vi "Main.vi"(8 "error in (no error)":errorcluster, 11 "AOTFBase in":refnum<class "AOTF.lvclass">) -> (0 "error out":errorcluster, 3 "component":refnum<class "AOTF.lvclass">)   [LabVIEW 2012, in "AOTF.lvclass"]
doc: "Main VI of the component."
uses:
  AOTF.lvclass
  <vilib>/Distrio/Murmex/Murmex/command_enum.ctl
  Controls/laser line ring.ctl
  <vilib>/Distrio/Murmex/InitialiseMessage/InitialiseMessage.lvclass
  AOTF.lvclass/AOTF.ctl
  <vilib>/Distrio/Murmex/ConfigureMessage/ConfigureMessage.lvclass
  <vilib>/Distrio/Murmex/TerminateMessage/TerminateMessage.lvclass
  <vilib>/Distrio/Murmex/Murmex/update_cluster.ctl
  <vilib>/Distrio/Murmex/Murmex/Set configure at initialise.vi
  <vilib>/Distrio/Murmex/Murmex/Set VI reference.vi
  <vilib>/Distrio/Murmex/Murmex/Get ID.vi
  <vilib>/Distrio/Murmex/Murmex/Set log reference.vi
  <vilib>/Distrio/Murmex/Murmex/Murmex.lvclass
  <vilib>/Distrio/Murmex/Message/Message.lvclass
panel:
  in  "button::configure":bool
  in  "button::quit":bool
  out "terminate?":bool=TRUE
  in  "Tab Control":enum32{"Main", "Debug"}(tab)
  in  "Power":dbl(knob) caption="Power [%]" min=0.0 max=100.0 scale=0.0..100.0
  in  "Wavelength":T1=10 items=["Blind"=10, "405nm"=0, "445nm"=5, "491nm"=1, "515nm"=2, "561nm"=3]
  out "log":string="\r\n11:11:41.970 05/12/2013: initialise from AOTF to AOTF\r\n11:11:42.586 05/12/2013: inform from AOTF to AOTF\r\n11:11:43.913 05/12/2013: update from AOTF to AOTF\r\n11:11:45.142 05/12/2013: generic (shutter_off) from AOTF to AOTF\r\n11:11:45.270 05/12/2013: generic (shutter_on) from AOTF to AOTF\r\n11:11:45.902 05/12/2013: generic (shutter_off) from AOTF to AOTF\r\n11:11:45.932 05/12/2013: inspect from AOTF to AOTF\r\n11:11:48.013 05/12/2013: configure from AOTF to AOTF\r\n11:11:52.003 05/12/2013: inform from AOTF to AOTF\r\n11:11:58.521 05/12/2013: initialise from AOTF to AOTF\r\n11:11:58.561 05/12/2013: inform from AOTF to AOTF\r\n11:11:58.695 05/12/2013: inform from AOTF to AOTF\r\n11:12:02.089 05/12/2013: update from AOTF to AOTF\r\n11:12:02.308 05/12/2013: inspect from AOTF to AOTF\r\n11:12:02.364 05/12/2013: inform from AOTF to AOTF\r\n11:12:05.062 05/12/2013: generic (shutter_on) from AOTF to AOTF\r\n11:12:06.690 05/12/2013: update from AOTF to AOTF\r\n11:12:06.909 05/12/2013: inspect from AOTF to AOTF\r\n11:12:06.964 05/12/2013: inform from AOTF to AOTF\r\n11:12:07.770 05/12/2013: update from AOTF to AOTF\r\n11:12:07.989 05/12/2013: inspect from AOTF to AOTF\r\n11:12:08.044 05/12/2013: inform from AOTF to AOTF\r\n11:12:08.627 05/12/2013: update from AOTF to AOTF\r\n11:12:08.846 05/12/2013: inspect from AOTF to AOTF\r\n11:12:08.900 05/12/2013: inform from AOTF to AOTF\r\n11:12:09.290 05/12/2013: update from AOTF to AOTF\r\n11:12:09.508 05/12/2013: inspect from AOTF to AOTF\r\n11:12:09.563 05/12/2013: inform from AOTF to AOTF\r\n11:12:10.154 05/12/2013: update from AOTF to AOTF\r\n11:12:10.373 05/12/2013: inspect from AOTF to AOTF\r\n11:12:10.430 05/12/2013: inform from AOTF to AOTF\r\n11:12:20.953 05/12/2013: update from AOTF to AOTF\r\n11:12:21.172 05/12/2013: inspect from AOTF to AOTF\r\n11:12:21.227 05/12/2013: inform from AOTF to AOTF\r\n11:12:22.057 05/12/2013: update from AOTF to AOTF\r\n11:12:22.276 05/12/2013: inspect from AOTF to AOTF\r\n11:12:22.330 05/12/2013: inform from AOTF to AOTF\r\n11:12:22.841 05/12/2013: update from AOTF to AOTF\r\n11:12:23.060 05/12/2013: inspect from AOTF to AOTF\r\n11:12:23.114 05/12/2013: inform from AOTF to AOTF\r\n11:12:23.449 05/12/2013: update from AOTF to AOTF\r\n11:12:23.668 05/12/2013: inspect from AOTF to AOTF\r\n11:12:23.724 05/12/2013: inform from AOTF to AOTF\r\n11:12:24.514 05/12/2013: update from AOTF to AOTF\r\n11:12:24.733 05/12/2013: inspect from AOTF to AOTF\r\n11:12:24.789 05/12/2013: inform from AOTF to AOTF\r\n11:12:25.098 05/12/2013: update from AOTF to AOTF\r\n11:12:25.317 05/12/2013: inspect from AOTF to AOTF\r\n11:12:25.371 05/12/2013: inform from AOTF to AOTF\r\n11:12:26.482 05/12/2013: update from AOTF to AOTF\r\n11:12:26.701 05/12/2013: inspect from AOTF to AOTF\r\n11:12:26.755 05/12/2013: inform from AOTF to AOTF\r\n11:12:27.154 05/12/2013: update from AOTF to AOTF\r\n11:12:27.373 05/12/2013: inspect from AOTF to AOTF\r\n11:12:27.428 05/12/2013: inform from AOTF to AOTF\r\n11:12:27.666 05/12/2013: update from AOTF to AOTF\r\n11:12:27.885 05/12/2013: inspect from AOTF to AOTF\r\n11:12:27.944 05/12/2013: inform from AOTF to AOTF\r\n11:12:33.380 05/12/2013: update from AOTF to AOTF\r\n11:12:33.484 05/12/2013: update from AOTF to AOTF\r\n11:12:33.603 05/12/2013: inspect from AOTF to AOTF\r\n11:12:33.611 05/12/2013: update from AOTF to AOTF\r\n11:12:33.684 05/12/2013: update from AOTF to AOTF\r\n11:12:33.740 05/12/2013: update from AOTF to AOTF\r\n11:12:33.827 05/12/2013: inspect from AOTF to AOTF\r\n11:12:33.835 05/12/2013: update from AOTF to AOTF\r\n11:12:33.897 05/12/2013: inform from AOTF to AOTF\r\n11:12:33.903 05/12/2013: update from AOTF to AOTF\r\n11:12:33.940 05/12/2013: update from AOTF to AOTF\r\n11:12:34.085 05/12/2013: update from AOTF to AOTF\r\n11:12:34.119 05/12/2013: inspect from AOTF to AOTF\r\n11:12:34.292 05/12/2013: update from AOTF to AOTF\r\n11:12:34.336 05/12/2013: inspect from AOTF to AOTF\r\n11:12:34.553 05/12/2013: inspect from AOTF to AOTF\r\n11:12:34.608 05/12/2013: inform from AOTF to AOTF\r\n11:12:34.739 05/12/2013: update from AOTF to AOTF\r\n11:12:34.771 05/12/2013: update from AOTF to AOTF\r\n11:12:34.826 05/12/2013: inspect from AOTF to AOTF\r\n11:12:34.834 05/12/2013: update from AOTF to AOTF\r\n11:12:34.867 05/12/2013: update from AOTF to AOTF\r\n11:12:34.931 05/12/2013: update from AOTF to AOTF\r\n11:12:34.979 05/12/2013: update from AOTF to AOTF\r\n11:12:35.003 05/12/2013: update from AOTF to AOTF\r\n11:12:35.027 05/12/2013: update from AOTF to AOTF\r\n11:12:35.041 05/12/2013: update from AOTF to AOTF\r\n11:12:35.051 05/12/2013: inspect from AOTF to AOTF\r\n11:12:35.066 05/12/2013: update from AOTF to AOTF\r\n11:12:35.116 05/12/2013: update from AOTF to AOTF\r\n11:12:35.171 05/12/2013: update from AOTF to AOTF\r\n11:12:35.211 05/12/2013: update from AOTF to AOTF\r\n11:12:35.273 05/12/2013: inspect from AOTF to AOTF\r\n11:12:35.287 05/12/2013: update from AOTF to AOTF\r\n11:12:35.475 05/12/2013: update from AOTF to AOTF\r\n11:12:35.495 05/12/2013: inspect from AOTF to AOTF\r\n11:12:35.549 05/12/2013: inform from AOTF to AOTF\r\n11:12:35.764 05/12/2013: inspect from AOTF to AOTF\r\n11:12:35.819 05/12/2013: inform from AOTF to AOTF\r\n11:12:35.861 05/12/2013: update from AOTF to AOTF\r\n11:12:35.877 05/12/2013: inform from AOTF to AOTF\r\n11:12:35.947 05/12/2013: update from AOTF to AOTF\r\n11:12:36.067 05/12/2013: update from AOTF to AOTF\r\n11:12:36.100 05/12/2013: inspect from AOTF to AOTF\r\n11:12:36.235 05/12/2013: update from AOTF to AOTF\r\n11:12:36.317 05/12/2013: inspect from AOTF to AOTF\r\n11:12:36.371 05/12/2013: inform from AOTF to AOTF\r\n11:12:36.587 05/12/2013: inspect from AOTF to AOTF\r\n11:12:36.771 05/12/2013: update from AOTF to AOTF\r\n11:12:36.804 05/12/2013: inspect from AOTF to AOTF\r\n11:12:37.020 05/12/2013: inspect from AOTF to AOTF\r\n11:12:37.238 05/12/2013: inspect from AOTF to AOTF\r\n11:12:37.456 05/12/2013: inspect from AOTF to AOTF\r\n11:12:37.673 05/12/2013: inspect from AOTF to AOTF\r\n11:12:37.891 05/12/2013: inspect from AOTF to AOTF\r\n11:12:37.946 05/12/2013: inform from AOTF to AOTF\r\n11:12:38.161 05/12/2013: inspect from AOTF to AOTF\r\n11:12:38.379 05/12/2013: inspect from AOTF to AOTF\r\n11:12:38.597 05/12/2013: inspect from AOTF to AOTF\r\n11:12:38.815 05/12/2013: inspect from AOTF to AOTF\r\n11:12:38.871 05/12/2013: inform from AOTF to AOTF\r\n11:12:39.086 05/12/2013: inspect from AOTF to AOTF\r\n11:12:39.303 05/12/2013: inspect from AOTF to AOTF\r\n11:12:39.363 05/12/2013: inform from AOTF to AOTF\r\n11:12:39.417 05/12/2013: inform from AOTF to AOTF\r\n11:12:39.633 05/12/2013: inspect from AOTF to AOTF\r\n11:12:39.852 05/12/2013: inspect from AOTF to AOTF\r\n11:12:40.069 05/12/2013: inspect from AOTF to AOTF\r\n11:12:40.124 05/12/2013: inform from AOTF to AOTF\r\n11:12:40.339 05/12/2013: inspect from AOTF to AOTF\r\n11:12:40.395 05/12/2013: inform from AOTF to AOTF\r\n11:12:40.448 05/12/2013: inform from AOTF to AOTF\r\n11:12:40.663 05/12/2013: inspect from AOTF to AOTF\r\n11:12:40.718 05/12/2013: inform from AOTF to AOTF\r\n11:12:40.770 05/12/2013: inform from AOTF to AOTF\r\n11:12:40.824 05/12/2013: inform from AOTF to AOTF\r\n11:12:40.877 05/12/2013: inform from AOTF to AOTF\r\n11:12:40.930 05/12/2013: inform from AOTF to AOTF\r\n11:12:40.982 05/12/2013: inform from AOTF to AOTF\r\n11:12:41.034 05/12/2013: inform from AOTF to AOTF\r\n11:12:41.092 05/12/2013: inform from AOTF to AOTF\r\n11:12:41.144 05/12/2013: inform from AOTF to AOTF\r\n11:12:41.196 05/12/2013: inform from AOTF to AOTF\r\n11:12:41.249 05/12/2013: inform from AOTF to AOTF\r\n11:12:41.307 05/12/2013: inform from AOTF to AOTF\r\n11:12:41.366 05/12/2013: inform from AOTF to AOTF\r\n11:12:41.424 05/12/2013: inform from AOTF to AOTF\r\n11:12:41.478 05/12/2013: inform from AOTF to AOTF\r\n11:12:41.533 05/12/2013: inform from AOTF to AOTF\r\n11:12:41.589 05/12/2013: inform from AOTF to AOTF\r\n11:12:42.246 05/12/2013: terminate from AOTF to AOTF"
  in  "component ID":string="AOTF"
  in  "button::send":bool
  in  "command":T2
  in  "Generic command":string
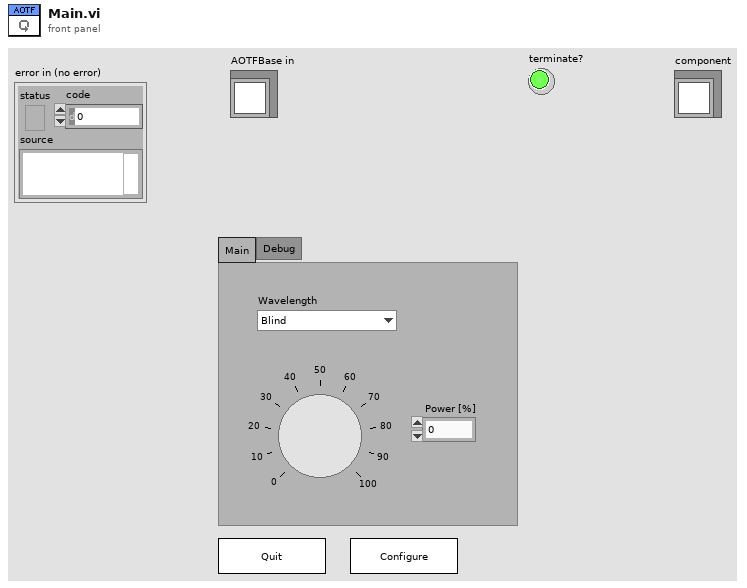
[diagram p1: front panel]
types:
  T1 = typedef "AOTF.lvclass/laser line ring.ctl" = u8
  T2 = typedef "Murmex.lvlib/Murmex.lvclass/command_enum.ctl" = enum16{"null", "initialise", "reset", "terminate", "acknowledge", "update", "inspect", "inform", "proceed", "start", "stop", "fetch", "configure", "generic"}
  T3 = enum8{"Enabled", "Disabled", "Disabled and Grayed Out"}
  T4 = typedef "Murmex.lvlib/Murmex.lvclass/update_cluster.ctl" = cluster{"target ID":string, "key chains":string[], "values":variant[]}
  T5 = typedef "Murmex.lvclass/command_enum.ctl" = enum16{"null", "initialise", "reset", "terminate", "acknowledge", "update", "inspect", "inform", "proceed", "start", "stop", "fetch", "configure", "generic"}
  T6 = typedef "Murmex.lvclass/Event type enumerations.ctl" = enum16{"before", "after"}
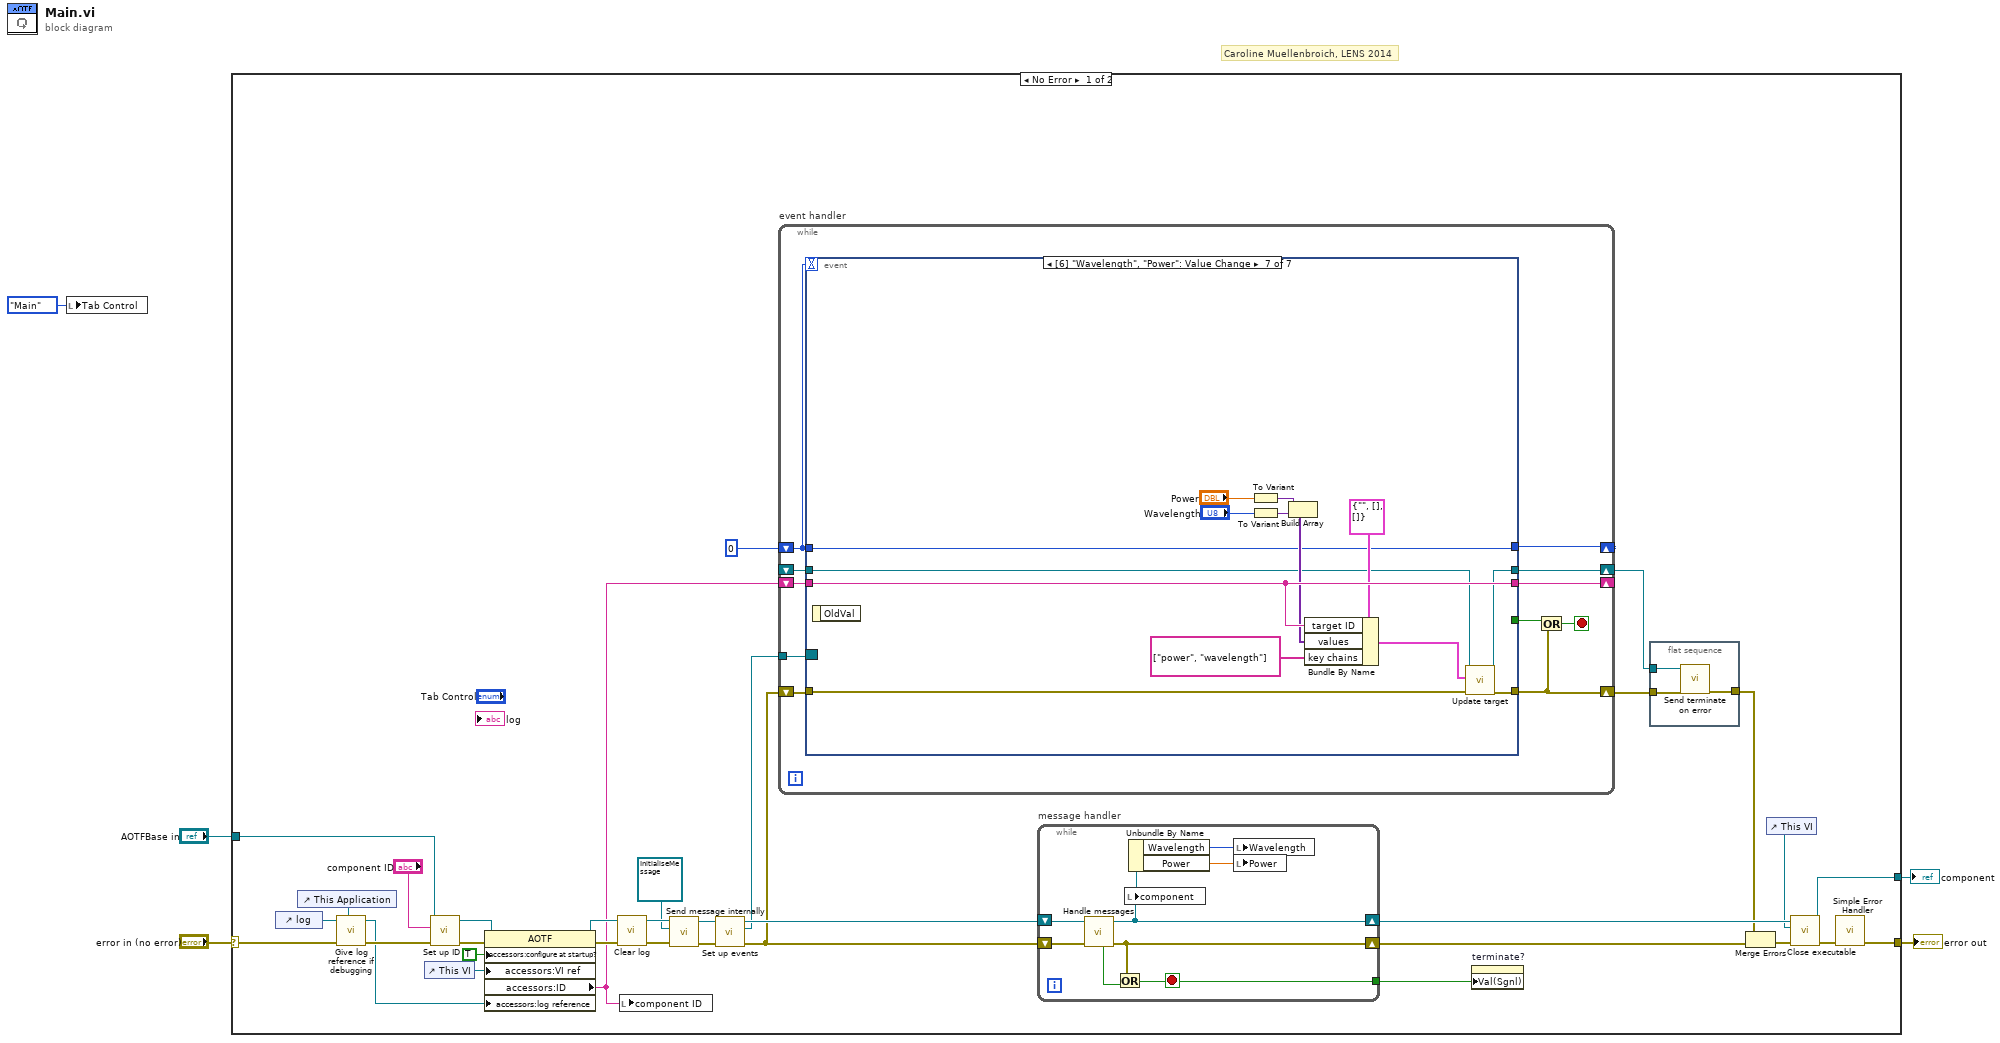
[diagram p0: block diagram]
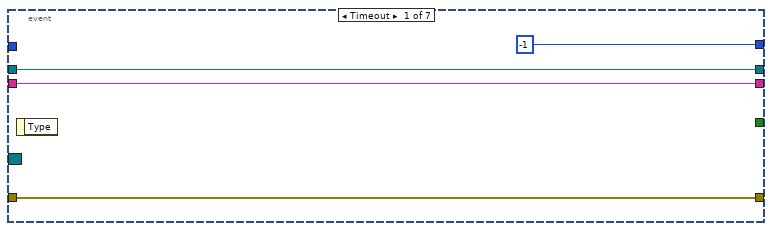
[diagram p2: hidden frame]
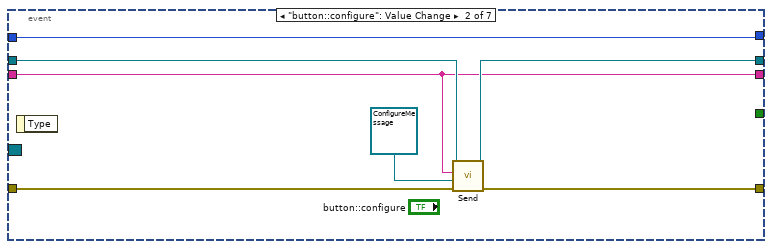
[diagram p3: hidden frame]
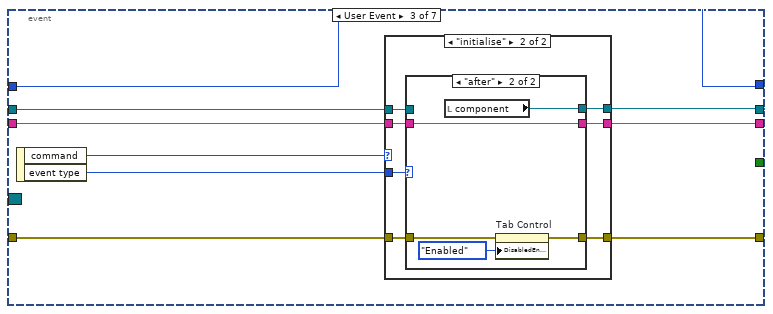
[diagram p4: hidden frame]
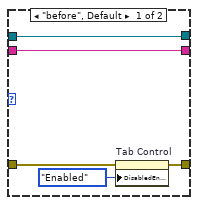
[diagram p6: hidden frame]
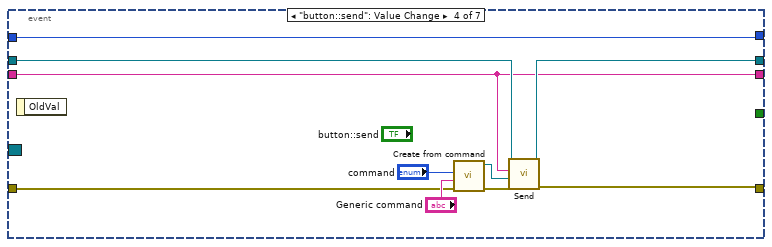
[diagram p7: hidden frame]
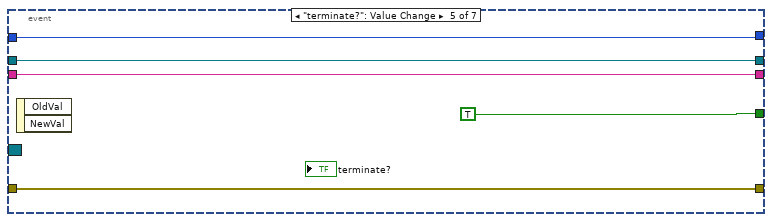
[diagram p8: hidden frame]
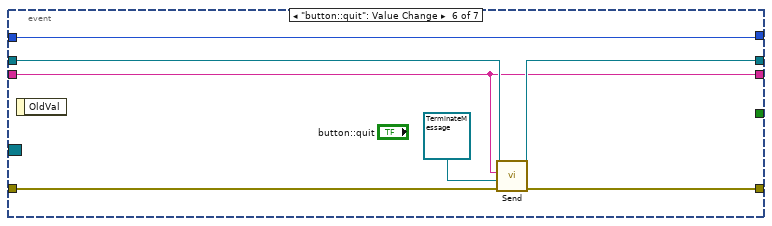
[diagram p9: hidden frame]
diagram:
  # "Caroline Muellenbroich, LENS 2014"
  n1 = local write "Tab Control"(enum32{"Main", "Debug"}."Main" ("Tab Control")) -> ()
  n2 = case shown="No Error" "error in (no error)" {
    selector: "error in (no error)" -> [w9 w139]
    tunnel: "AOTFBase in" -> [w39 w138]
    tunnel: [w24 w138] -> w5
    tunnel: [w20 w139] -> w4
    frame No Error {
      n3 = control-ref of="log"() -> (w10:refnum<vi>)
      n4 = control-ref of="This Application"() -> (w11:refnum<vi>)
      n5 = call "Give log reference if debugging.vi"("application ref"=w11, "error in (no error)"=w9, "log reference in"=w10) -> ("error out"=w8:errorcluster, "log reference out"=w7:refnum<vi>)  [unwired: 6 in, 1 out]
      n6 = control-ref of="This VI"() -> (w35:refnum<vi>)
      n7 = call <vilib>:"Set up ID.vi"("error in (no error)"=w8, "component ID"="component ID", "MurmexBase in"=w39) -> ("error out"=w38:errorcluster, "MurmexBase out"=w37:refnum<class "AOTF.lvclass">)  [unwired: 6 in, 1 out]
      n8 = property class="AOTF"(reference=w37, error in=w38, "accessors:configure at startup?"=TRUE ("configure at startup?"), "accessors:VI ref"=w35, "accessors:log reference"=w7) -> (reference out=w32:refnum<class "AOTF.lvclass">, error out=w34:errorcluster, "accessors:ID"=w14:string)
      n9 = call <vilib>:"Clear log.vi"("error in (no error)"=w34, "MurmexBase in"=w32) -> ("error out"=w33:errorcluster, "MurmexBase out"=w31:refnum<class "AOTF.lvclass">)  [unwired: 8 in]
      n10 = local write "component ID"(w14) -> ()
      n11 = call <vilib>:"Send message internally.vi"("error in (no error)"=w33, "Message"=refnum<class "InitialiseMessage.lvclass"> refnum ("Murmex.lvlib:InitialiseMessage"), "Murmex in"=w31) -> ("error out"=w30:errorcluster, "Murmex out"=w6:refnum<class "AOTF.lvclass">)  [unwired: 7 in]
      n12 = call <vilib>:"Set up events.vi"("error in (no error)"=w30, "MurmexBase in"=w6) -> ("error out"=w23:errorcluster, "Event Registration Refnum"=w22:refnum<event-registration>, "MurmexBase out"=w29:refnum<class "AOTF.lvclass">)  [unwired: 7 in]
      n13 = while "event handler" {
        tunnel: w22 -> [w53]
        shift-right: [w46] -> w18
        shift-left: w23 -> [w52]
        shift-right: [w48] -> _
        shift-left: w14 -> [w51]
        shift-right: [w50] -> w16
        shift-left: _ -> [w49]
        shift-right: [w44] -> _
        shift-left: 0 -> [w43]
        stop <- w47 stop-if-true
        n14 = event shown="[6] \"Wavelength\", \"Power\": Value Change" {
          selector: w53 -> [_ _ _ _ _ _ _]
          dyn-events: _ -> [_ _ _ _ _ _ _]
          timeout: w43 -> [_ _ _ _ _ _ _]
          tunnel: w52 -> [w55 w64 w71 w100 w108 w115 w128]
          tunnel: [w55 w63 w70 w99 w108 w114 w129] -> w46
          tunnel: w51 -> [w57 w59 w69 w95 w106 w110 w127]
          tunnel: [w56 w61 w68 w97 w105 w112 w122] -> w50
          tunnel: w49 -> [w56 w62 w67 w98 w105 w113 w118]
          tunnel: [w57 w59 w66 w95 w106 w110 w127] -> w48
          tunnel: [_ _ _ _ TRUE _ _] -> w45
          tunnel: w43 -> [_ w60 w65 w96 w104 w111 w119]
          tunnel: [-1 w60 w65 w96 w104 w111 w119] -> w44
          event Timeout {
            n15 = event-data() -> ()  [unwired: 1 in, 1 out]
          }
          event "button::configure": Value Change {
            n16 = event-data() -> ()  [unwired: 1 in, 1 out]
            n17 = call <vilib>:"Send.vi"("error in (no error)"=w64, "Message"=refnum<class "ConfigureMessage.lvclass"> refnum ("Murmex.lvlib:ConfigureMessage"), "recipient"=w59, "Murmex in"=w62) -> ("error out"=w63:errorcluster, "Murmex out"=w61:refnum<class "AOTF.lvclass">)  [unwired: 6 in]
          }
          event User Event {
            n18 = event-data() -> ("command"=w73:T5, "event type"=w72:T6)  [unwired: 1 in]
            n19 = case shown="\"initialise\"" w73 {
              tunnel: w72 -> [_ w83]
              tunnel: w71 -> [w74 w82]
              tunnel: [w74 w81] -> w70
              tunnel: w69 -> [w76 w80]
              tunnel: [w75 w79] -> w68
              tunnel: w67 -> [w75 w78]
              tunnel: [w76 w77] -> w66
              frame "null", Default {
              }
              frame "initialise" {
                n20 = case shown="\"after\"" w83 {
                  tunnel: [w87 w92] -> w81
                  tunnel: w82 -> [w88 w93]
                  tunnel: w80 -> [w85 w90]
                  tunnel: [w84 w89] -> w79
                  tunnel: w78 -> [w84 _]
                  tunnel: [w85 w90] -> w77
                  frame "before", Default {
                    n21 = property on="Tab Control" class="TabCtl (strict)"(error in=w88, "DisabledEnum"=T3."Enabled" ("Disabled")) -> (error out=w87:errorcluster)  [unwired: 1 in, 1 out]
                  }
                  frame "after" {
                    n22 = local read "component"() -> (w89:refnum<class "AOTF.lvclass">)
                    n23 = property on="Tab Control" class="TabCtl (strict)"(error in=w93, "DisabledEnum"=T3."Enabled" ("Disabled")) -> (error out=w92:errorcluster)  [unwired: 1 in, 1 out]
                  }
                }
              }
            }
          }
          event "button::send": Value Change {
            n24 = event-data() -> ()  [unwired: 1 in, 1 out]
            n25 = call <vilib>:"Create from command.vi"("error in (no error)"=w100, "generic command"="Generic command", "command"="command") -> ("error out"=w102:errorcluster, "Message out"=w101:refnum<class "Message.lvclass">)  [unwired: 7 in]
            n26 = call <vilib>:"Send.vi"("error in (no error)"=w102, "Message"=w101, "recipient"=w95, "Murmex in"=w98) -> ("error out"=w99:errorcluster, "Murmex out"=w97:refnum<class "AOTF.lvclass">)  [unwired: 6 in]
          }
          event "terminate?": Value Change {
            n27 = event-data() -> ()  [unwired: 1 in, 2 out]
          }
          event "button::quit": Value Change {
            n28 = event-data() -> ()  [unwired: 1 in, 1 out]
            n29 = call <vilib>:"Send.vi"("error in (no error)"=w115, "Message"=refnum<class "TerminateMessage.lvclass"> refnum ("Murmex.lvlib:TerminateMessage"), "recipient"=w110, "Murmex in"=w113) -> ("error out"=w114:errorcluster, "Murmex out"=w112:refnum<class "AOTF.lvclass">)  [unwired: 6 in]
          }
          event "Power": Value Change {
            n30 = event-data() -> ()  [unwired: 1 in, 1 out]
            n31 = To Variant(anything="Power") -> (Variant=w121:variant)
            n32 = To Variant(anything="Wavelength") -> (Variant=w120:variant)
            n33 = Build Array(w121, w120) -> (w123:variant[])
            n34 = Bundle By Name(cluster=T4 {"target ID"="", "key chains"=[], "values"=[]} ("update cluster"), "target ID"=w127, "values"=w123, "key chains"=string[] ["power", "wavelength"]) -> (w126:T4)
            n35 = call <vilib>:"Update target.vi"("error in (no error)"=w128, "update cluster"=w126, "MurmexBase in"=w118) -> ("error out"=w129:errorcluster, "MurmexBase out"=w122:refnum<class "AOTF.lvclass">)  [unwired: 7 in]
          }
        }
        n36 = Or(x=w45, y=w46) -> (x .or. y?=w47:bool)
      }
      n37 = while "message handler" {
        shift-right: [w132] -> w25
        shift-left: w29 -> [w136]
        shift-right: [w135] -> w26
        shift-left: w23 -> [w137]
        tunnel: [w133] -> w21
        stop <- w133 stop-if-true
        n38 = call <vilib>:"Handle messages.vi"("error in (no error)"=w137, "Murmex in"=w136) -> ("error out"=w135:errorcluster, "Murmex out"=w132:refnum<class "AOTF.lvclass">, "terminated?"=w134:bool)  [unwired: 7 in]
        n39 = Or(x=w135, y=w134) -> (x .or. y?=w133:bool)
        n40 = local write "component"(w132) -> ()
        n41 = Unbundle By Name(w132) -> ("Wavelength"=w130:T1, "Power"=w131:dbl)
        n42 = local write "Wavelength"(w130) -> ()
        n43 = local write "Power"(w131) -> ()
      }
      n44 = property on="terminate?" class="Bool (strict)"("Val(Sgnl)"=w21) -> ()  [unwired: 2 in, 2 out]
      n45 = flat-sequence {
        tunnel: w18 -> [w41]
        tunnel: [w42] -> w17
        tunnel: w16 -> [w40]
        frame #0 {
          n46 = call <vilib>:"Send terminate on error.vi"("error in (no error)"=w41, "Murmex in"=w40) -> ("error out"=w42:errorcluster)  [unwired: 8 in, 1 out]
        }
      }
      n47 = Merge Errors(w17, w26) -> (w27:errorcluster)
      n48 = control-ref of="This VI"() -> (w15:refnum<vi>)
      n49 = call <vilib>:"Close executable.vi"("error in (no error)"=w27, "main VI ref (optional)"=w15, "MurmexBase in"=w25) -> ("error out"=w28:errorcluster, "MurmexBase out"=w24:refnum<class "AOTF.lvclass">)  [unwired: 7 in]
      n50 = call <vilib>:"Simple Error Handler.vi"("error in (no error)"=w28) -> ("error out"=w20:errorcluster)  [unwired: 4 in, 4 out]
    }
    frame Error {
    }
  }
  "error out" <- w4
  "component" <- w5
